vi "Humidity Write.vi"   [LabVIEW 2023, in "Climate Chamber.lvclass"]
uses:
  Climate Chamber.lvclass
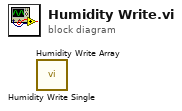
[diagram p0: block diagram]
diagram:
  n1 = call "Humidity Write Single.vi"() -> ()  [unwired: 10 in, 2 out]
  n2 = call "Humidity Write Array.vi"() -> ()  [unwired: 10 in, 2 out]
